vi "Status Channel.vi"(8 "error in (no error)":errorcluster, 11 "Node Ptr":T1 format="%.0x") -> (0 "error out":errorcluster)   [LabVIEW 2020, in "Ballard ARINC 429 System Explorer.lvlib" / "Implementation.lvlib"]
uses:
  Implementation.lvlib
  <vilib>/NI VeriStand/Custom Device API/Custom Device Item Ref.ctl
  <vilib>/NI VeriStand/Custom Device API/Custom Device API.lvlib
panel:
  in  "General Header":cluster{"Section Name":string}={"Section Name"="Ballard ARINC 429 - Status Channel"}
  out "Name":string
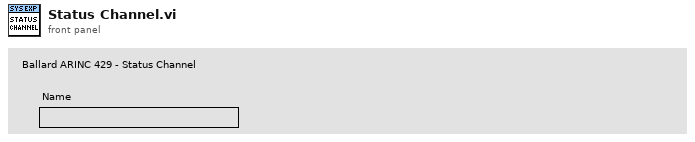
[diagram p1: front panel]
types:
  T1 = typedef "Custom Device API.lvlib/Custom Device Item Ref.ctl" = u64
  T2 = typedef "Custom Device API.lvlib/Custom Device Item Info.ctl" = cluster{"Name":string, "Is Channel":bool, "GUID":string, "Is Waveform":bool}
  T3 = typedef "Custom Device API.lvlib/Custom Device Commands.ctl" = enum16{"Default", "Item renamed", "Shutdown", "Dynamic button pressed"}
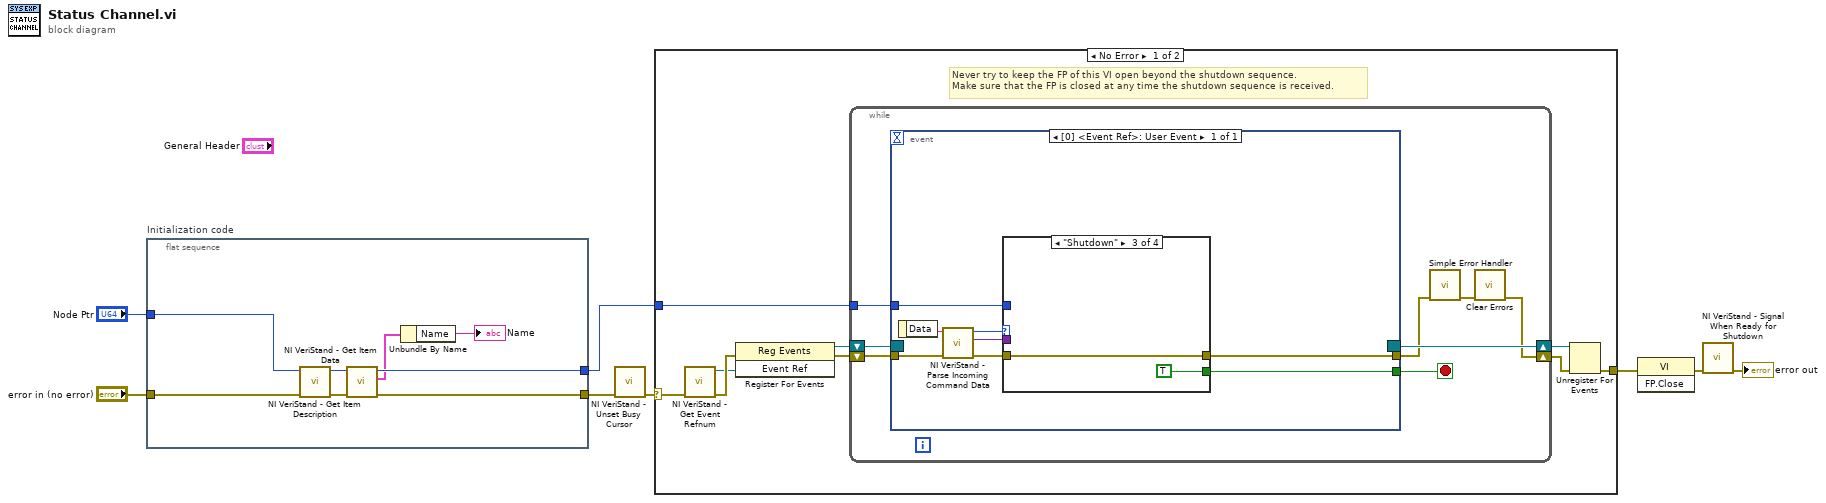
[diagram p0: block diagram]
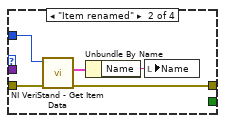
[diagram p3: hidden frame]
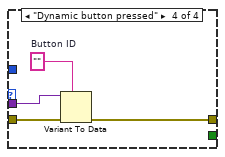
[diagram p4: hidden frame]
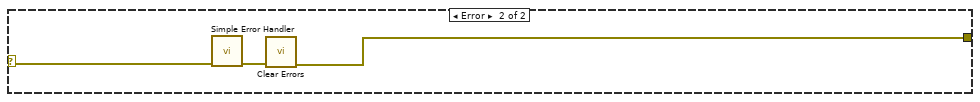
[diagram p5: hidden frame]
diagram:
  n1 = flat-sequence "Initialization code" {
    tunnel: "error in (no error)" -> [w10]
    tunnel: "Node Ptr" -> [w11]
    tunnel: [w12] -> w4
    tunnel: [w16] -> w1
    frame #0 {
      n2 = call <vilib>:"NI VeriStand - Get Item Description.vi"("error in (no error)"=w10, "Item Ref in"=w11) -> ("error out"=w14:errorcluster, "Item Ref out"=w15:T1)  [unwired: 8 out]
      n3 = call <vilib>:"NI VeriStand - Get Item Data.vi"("error in (no error)"=w14, "Item Ref in"=w15) -> ("error out"=w12:errorcluster, "Item Info"=w13:T2, "Item Ref out"=w16:T1)  [unwired: 7 out]
      n4 = Unbundle By Name(w13) -> ("Name"=→"Name":string)
    }
  }
  n5 = call <vilib>:"NI VeriStand - Unset Busy Cursor.vi"("error in (no error)"=w4) -> ("error out"=w3:errorcluster)  [unwired: 10 out]
  n6 = case shown="No Error" w3 {
    selector: w3 -> [w17 w56]
    tunnel: [w22 w54] -> w8
    tunnel: w1 -> [w18 _]
    frame No Error {
      # "Never try to keep the FP of this VI open beyond the shutdown sequence.\nMake sure that the FP is closed at any time the shutdown sequence is received."
      n7 = call <vilib>:"NI VeriStand - Get Event Refnum.vi"("error in (no error)"=w17) -> ("error out"=w25:errorcluster, "Event Ref"=w21:refnum<user-event>)  [unwired: 9 out]
      n8 = register-events(error in=w25, w21) -> (reference out=w19:refnum<event-registration>, error out=w20:errorcluster)  [unwired: 1 in]
      n9 = while {
        tunnel: w18 -> [w29]
        shift-right: [w26] -> w23
        shift-left: w20 -> [w32]
        shift-right: [w33] -> w24
        shift-left: w19 -> [w31]
        stop <- w30 stop-if-true
        n10 = event shown="[0] <Event Ref>: User Event" {
          selector: w31 -> [_]
          dyn-events: [_] -> w33
          timeout: _ -> [_]
          tunnel: w32 -> [w41]
          tunnel: [w37] -> w30
          tunnel: [w36] -> w28
          tunnel: w29 -> [w35]
          event User Event {
            n11 = event-data() -> ("Data"=w40:string)  [unwired: 1 out]
            n12 = call <vilib>:"NI VeriStand - Parse Incoming Command Data.vi"("error in (no error)"=w41, "Incoming data"=w40) -> ("error out"=w39:errorcluster, "Outgoing data"=w34:variant, "Action"=w38:T3)  [unwired: 7 out]
            n13 = case shown="\"Shutdown\"" w38 {
              tunnel: w39 -> [w42 w47 w48 w53]
              tunnel: [_ _ TRUE _] -> w37
              tunnel: [w42 w44 w48 w50] -> w36
              tunnel: w35 -> [_ w46 _ _]
              tunnel: w34 -> [_ _ _ w52]
              frame "Default", Default {
              }
              frame "Item renamed" {
                n14 = call <vilib>:"NI VeriStand - Get Item Data.vi"("error in (no error)"=w47, "Item Ref in"=w46) -> ("error out"=w44:errorcluster, "Item Info"=w45:T2)  [unwired: 8 out]
                n15 = Unbundle By Name(w45) -> ("Name"=w43:string)
                n16 = local write "Name"(w43) -> ()
              }
              frame "Shutdown" {
              }
              frame "Dynamic button pressed" {
                w51 = ""  # Button ID
                n17 = Variant To Data(error in=w53, type=w51, Variant=w52) -> (error out=w50:errorcluster)  [unwired: 1 out]
              }
            }
          }
        }
        n18 = call <vilib>:"Simple Error Handler.vi"("error in (no error)"=w28) -> ("error out"=w27:errorcluster)  [unwired: 1 in, 7 out]
        n19 = call <vilib>:"Clear Errors.vi"("error in (no error)"=w27) -> ("error out"=w26:errorcluster)  [unwired: 1 in, 5 out]
      }
      n20 = Unregister For Events(event registration refnum=w24, error in=w23) -> (error out=w22:errorcluster)
    }
    frame Error {
      n21 = call <vilib>:"Simple Error Handler.vi"("error in (no error)"=w56) -> ("error out"=w55:errorcluster)  [unwired: 1 in, 7 out]
      n22 = call <vilib>:"Clear Errors.vi"("error in (no error)"=w55) -> ("error out"=w54:errorcluster)  [unwired: 1 in, 5 out]
    }
  }
  n23 = invoke class="VI" method="FP.Close"(error in=w8) -> (error out=w7:errorcluster)  [unwired: 2 in, 2 out]
  n24 = call <vilib>:"NI VeriStand - Signal When Ready for Shutdown.vi"("error in (no error)"=w7) -> ("error out"=→"error out":errorcluster)  [unwired: 10 out]
